vi "From JSON.vi"(8 "error in (no error)":errorcluster, 10 "JSON":string, 11 "Double Float in":refnum<class "Abs_Complex Single Float 1D.lvclass">) -> (0 "error out":errorcluster, 3 "Double Float out":refnum<class "Abs_Complex Single Float 1D.lvclass">)   [LabVIEW 2021, in "Abs_Complex Single Float 1D.lvclass"]
uses:
  Abs_Complex Single Float 1D.lvclass
  C:/Program Files (x86)/National Instruments/LabVIEW 2021/vi.lib/TSA/Abstract Data Classes/Abs_Types/Type/Abs_Type.lvclass
  Support/Type.ctl
  8a4985c5-1e86-4595-bcc0-7f9c82563bff.vi
  <vilib>/JDP Science/JSONtext/Find Item.vi
  <vilib>/JDP Science/JSONtext/Next JSON Value.vi
  <vilib>/JDP Science/JSONtext/String Subset.vi
  <vilib>/JDP Science/JSONtext/Parsing/Advance past next JSON Value (inlined COPY).vi
  <vilib>/JDP Science/JSONtext/Parsing/Advance past whitespace.vi
  <vilib>/JDP Science/JSONtext/Parsing/Advance past String.vi
  <vilib>/JDP Science/JSONtext/Parsing/Advance past Number.vi
  <vilib>/JDP Science/JSONtext/Parsing/Advance past Line Ending.vi
  <vilib>/Utility/LVClass/Get LV Class Name.vi
  <vilib>/JDP Science/JSONtext/Parsing/Parse Full Path or Item Name.vi
  <vilib>/JDP Science/JSONtext/Parsing/Advance past Array.vi
  <vilib>/JDP Science/JSONtext/Parsing/Advance past Object.vi
  <vilib>/JDP Science/JSONtext/support/Error Cluster From Code.vi
  <vilib>/JDP Science/JSONtext/Offset/Find Item Locations by Path.vi
  <vilib>/JDP Science/JSONtext/JSON text to Variant.vi
  <vilib>/JDP Science/JSONtext/LVClass Serializer/JSONtext LVClass Serializer.lvclass
  Floating Point 1D/Abs_Floating Point 1D.lvclass
  Type/Abs_Type.lvclass
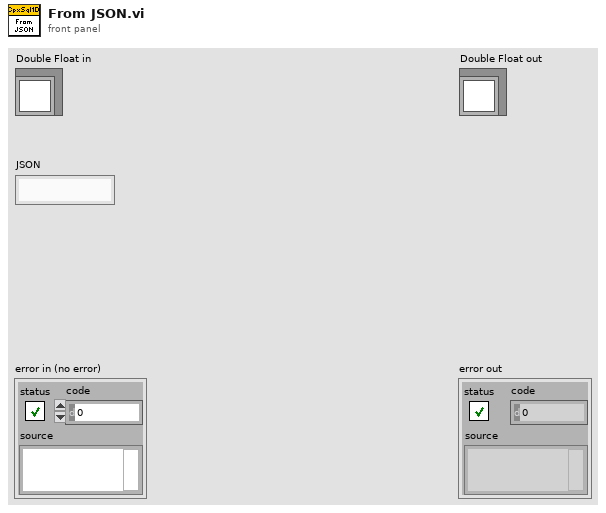
[diagram p1: front panel]
types:
  T1 = typedef "Abs_Complex Single Float 1D.lvclass/Type.ctl" = csg[]
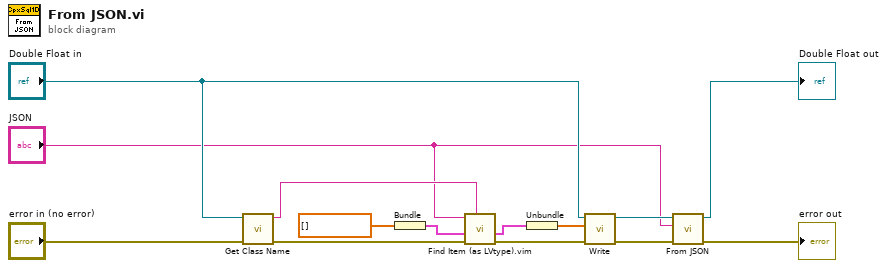
[diagram p0: block diagram]
diagram:
  n1 = call "Get Class Name.vi"("error in (no error)"="error in (no error)", "Abs_Type in"="Double Float in") -> ("error out"=w7:errorcluster, "class name"=w8:string)  [unwired: 8 in]
  n2 = Bundle("Value"=T1 []) -> (w9:cluster{"Value":T1})  [unwired: 1 in]
  n3 = call "Find Item (as LVtype).vim"("$Path or Item Name"=w8, "error in (no error)"=w7, "Data Type and Default Value"=w9, "JSON"="JSON") -> ("error out"=w6:errorcluster, "Data"=w10:cluster{"Value":T1})  [unwired: 4 in, 2 out]
  n4 = Unbundle(w10) -> ("Value"=w3:T1)
  n5 = call-dynamic "Write.vi"("error in (no error)"=w6, "Value"=w3, "Double Float.lvclass in"="Double Float in") -> ("error out"=w5:errorcluster, "Double Float.lvclass out"=w4:refnum<class "Abs_Complex Single Float 1D.lvclass">)  [unwired: 7 in]
  n6 = call-parent "From JSON.vi"("error in (no error)"=w5, "JSON"="JSON", "Type in"=w4) -> ("error out"=→"error out":errorcluster, "Type out"=→"Double Float out":refnum<class "Abs_Complex Single Float 1D.lvclass">)  [unwired: 7 in]
